vi "Example Interrupt - InputValue Callback.vi"(4 "InputValue":refnum<user-event>, 5 "Event Data":T1, 6 "Control Ref":refnum<k24>, 7 "Event Common Data":T2) -> ()   [LabVIEW 2013]
uses:
  C:/tf/play/labview/Tinkerforge.dll
  Tinkerforge.dll
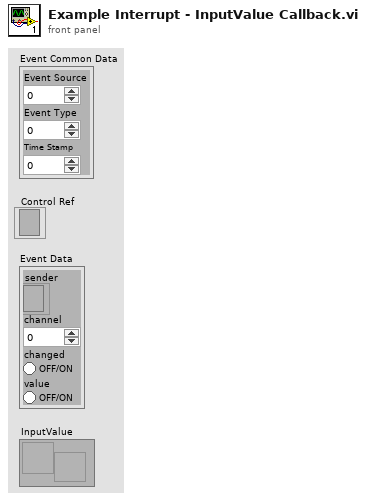
[diagram p1: front panel]
types:
  T1 = cluster{"sender":refnum<k24>, "channel":u8, "changed":bool, "value":bool}
  T2 = cluster{"Event Source":i32, "Event Type":u32, "Time Stamp":u32}
  T3 = cluster{"channel":u8, "changed":bool, "value":bool}
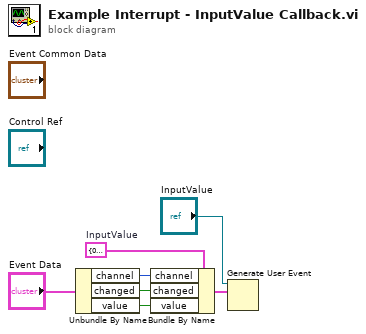
[diagram p0: block diagram]
diagram:
  w3 = T3 {"channel"=0, "changed"=FALSE, "value"=FALSE}  # InputValue
  n1 = Unbundle By Name("Event Data") -> ("channel"=w7:u8, "changed"=w6:bool, "value"=w2:bool)
  n2 = Bundle By Name(cluster=w3, "channel"=w7, "changed"=w6, "value"=w2) -> (w5:T3)
  n3 = Generate User Event(user event="InputValue", event data cluster=w5) -> ()  [unwired: 2 in, 2 out]
